vi "24_UNDT_Freq (SubVI).vi"(8 "error in":errorcluster, 10 "UNDT_Freq":i32, 11 "String in":refnum<vi>) -> (0 "error out":errorcluster)   [LabVIEW 2017]
uses:
  Global_SNK3_HF.vi
  E:/_git/LV_Unicorn/LV_Unicorn.lvlib
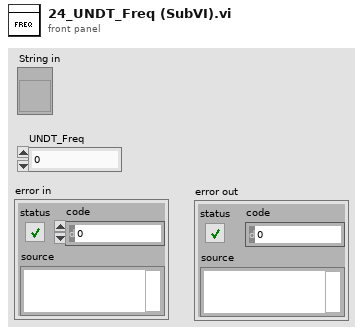
[diagram p1: front panel]
types:
  T1 = typedef "LV_Unicorn.lvlib/unicorn_Param.ctl" = cluster{"conParam":T2, "Param":T3}
  T2 = typedef "LV_Unicorn.lvlib/unicorn_conn.ctl" = cluster{"ReadIntParam":bool, "ReadDescrParam":bool, "ReadFloatParam":bool, "debug":bool, "ReadJSON":bool, "IP_address":string, "N_attempts":i32, "type_con":enum16{"Serial", "TCP"}, "MB_address":i32, "VISA":refnum<visa-resource-name>, "connection ID":refnum<k5>, "nameDevices":string, "timeout":i32, "port":u16, "type_version":string, "baud_rate":u32, "VersionControl":bool, "TCP_conn":bool, "WindowSize":i32}
  T3 = typedef "LV_Unicorn.lvlib/unicorn_JSON.ctl" = cluster{"NumParam":cluster{"NTelem":i32, "NInt":i32, "NFloat":i32, "NTable":i32}, "ParamInt":T4, "Telemetry":T5, "Table":T6, "ParamFloat":T7}
  T4 = typedef "LV_Unicorn.lvlib/unicorn_ParamInt.ctl" = cluster{"ID":string, "Num":i32, "Name":string, "Type":string, "Enum":string, "Desc":string, "Unit":string, "Access":string, "FormatStr":string, "Min":i32, "Max":i32}[]
  T5 = typedef "LV_Unicorn.lvlib/unicorn_Telemetry.ctl" = cluster{"ID":string, "Num":i32, "Name":string, "Desc":string, "Unit":string, "FormatStr":string, "Min":i32, "Max":i32}[]
  T6 = typedef "LV_Unicorn.lvlib/unicorn_Table.ctl" = cluster{"Num":i32, "Access":string, "ColumnCount":i32, "NeedParamPrepare":bool, "Columns":cluster{"Column":i32, "Desc":string, "Name":string}[], "DataType":string, "FormatStr":string, "ID":string, "Name":string, "RowCount":i32, "Rows":cluster{"Desc":string, "ID":string, "Max":i32, "Min":i32, "Name":string, "Row":i32, "Unit":string}[], "Type":string}[]
  T7 = typedef "LV_Unicorn.lvlib/unicorn_ParamFloat.ctl" = cluster{"ID":string, "Num":i32, "Name":string, "Type":string, "Enum":string, "Desc":string, "Unit":string, "Access":string, "FormatStr":string, "Min":sgl, "Max":sgl}[]
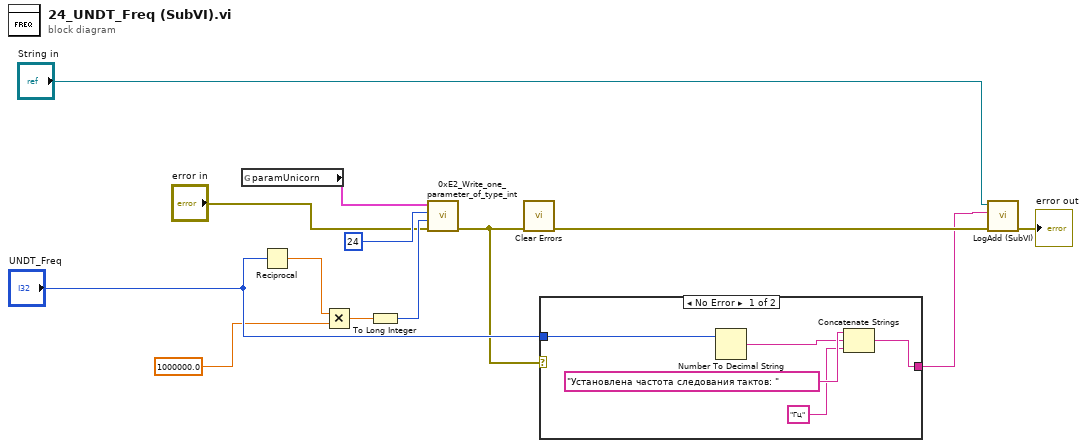
[diagram p0: block diagram]
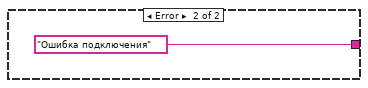
[diagram p2: hidden frame]
diagram:
  n1 = global read "Global_SNK3_HF.vi" "paramUnicorn"() -> (w10:T1)
  n2 = Reciprocal(x="UNDT_Freq") -> (1/x=w5:dbl)
  n3 = Multiply(x=w5, y=1000000.0) -> (x*y=w7:dbl)
  n4 = To Long Integer(number=w7) -> (32bit integer=w8:i32)
  n5 = call "0xE2_Write_one_parameter_of_type_int.vi"("error in"="error in", "ParamIn"=w8, "NumParamIn"=24 ("Номер параметра"), "paramUnicorn 2"=w10) -> ("error out"=w1:errorcluster)  [unwired: 4 in, 3 out]
  n6 = call <vilib>:"Clear Errors.vi"("error in (no error)"=w1) -> ("error out"=w13:errorcluster)  [unwired: 5 in, 1 out]
  n7 = case shown="No Error" w1 {
    tunnel: "UNDT_Freq" -> [w18 _]
    tunnel: [w15 "Ошибка подключения" ("t")] -> w12
    frame No Error {
      n8 = Number To Decimal String(number=w18) -> (decimal integer string=w16:string)  [unwired: 1 in]
      n9 = Concatenate Strings("Установлена частота следования тактов: " ("string"), w16, "Гц" ("string")) -> (w15:string)
    }
    frame Error {
    }
  }
  n10 = call "LogAdd (SubVI).vi"("error in"=w13, "string"=w12, "Log"="String in") -> ("error out"=→"error out":errorcluster)  [unwired: 8 in]
